vi "Prod_Screen.vi"(1 "gain_in":dbl format="%#_13g", 2 "nf_in":dbl format="%#_13g", 3 "pow_in":dbl format="%#_13g", 5 "error in (no error)":errorcluster, 7 "s11_in":dbl format="%#_13g", 9 "txflat_in":dbl format="%#_13g", 11 "pout_in":dbl format="%#_13g") -> (6 "rx_p-f":string, 8 "tx_p-f":string, 10 "RX-PASS?(T)":bool, 12 "TX-PASS?(T)":bool, 15 "prod_lim_p-f":string, 19 "error out":errorcluster)   [LabVIEW 2018]
uses:
  Tetra_Globals.vi
panel:
  out "gain_lsl":dbl
  out "names 10":string
  out "end":bool
  out "pout_pass?(t)":bool
  out "tx-flat_pass?(t)":bool
  out "s11_pass?(t)":bool
  out "pow_pass?(t)":bool
  out "nf_pass?(t)":bool
  out "gain_pass?(t)":bool
  out "names 9":string
  out "limits 9":dbl
  out "names 8":string
  out "limits 8":dbl
  out "names 7":string
  out "pout_hsl":dbl
  out "names 6":string
  out "pout_lsl":dbl
  out "names 5":string
  out "txflat":dbl
  out "names 4":string
  out "s11_hsl":dbl
  out "names 3":string
  out "pow_hsl":dbl
  out "names 2":string
  out "nf_hsl":dbl
  out "gain_hsl":dbl
  out "names":string
  # "pdc|g|nf"
  # "pdc|s11|txf|txp"
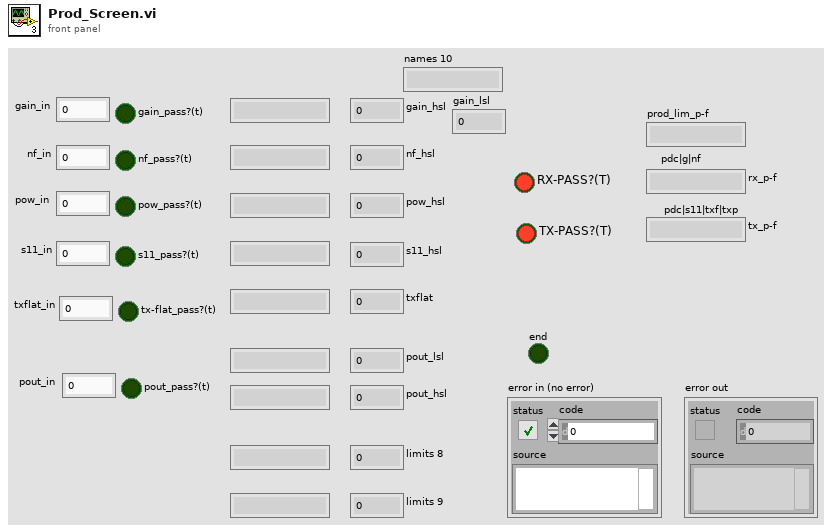
[diagram p1: front panel]
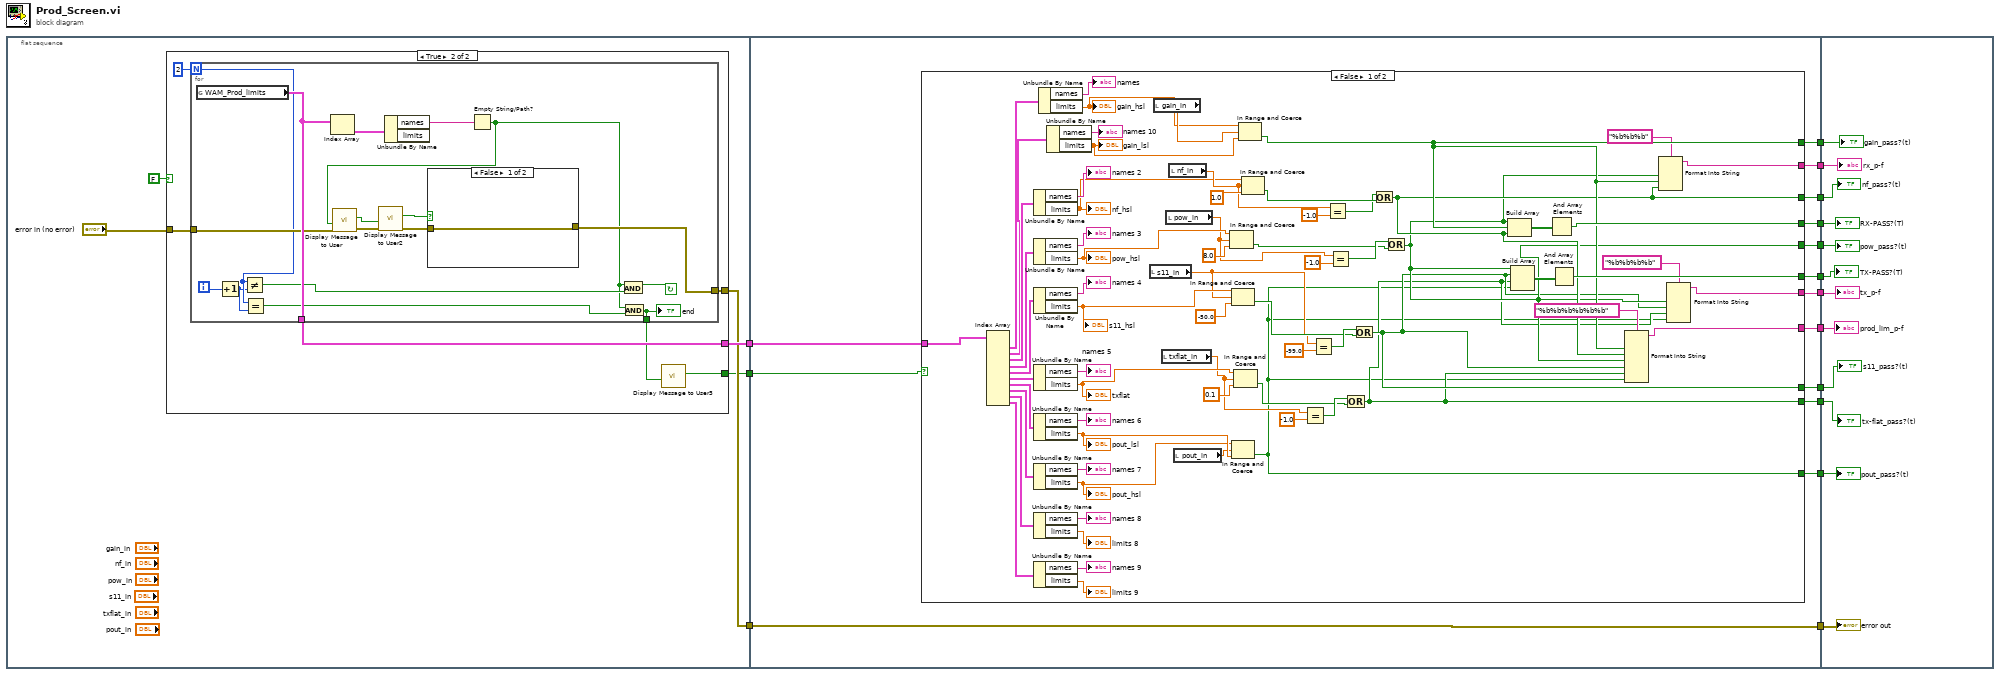
[diagram p0: block diagram]
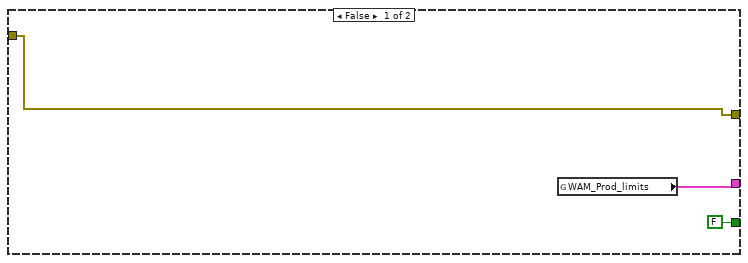
[diagram p2: hidden frame]
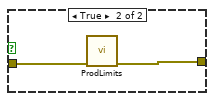
[diagram p3: hidden frame]
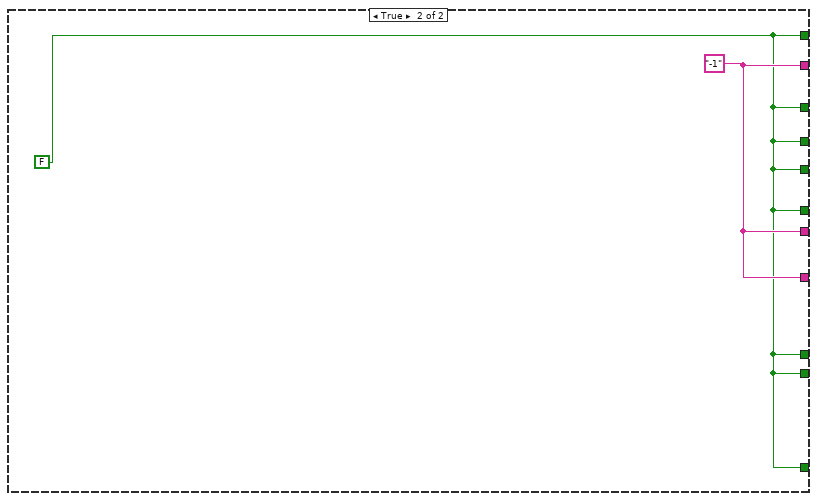
[diagram p4: hidden frame]
diagram:
  n1 = flat-sequence {
    tunnel: [w20] -> w15
    tunnel: [w18] -> w13
    tunnel: [w17] -> w12
    tunnel: w15 -> [w63]
    tunnel: [w62] -> w14
    tunnel: w13 -> [w62]
    tunnel: w12 -> [w61]
    tunnel: [w60] -> w11
    tunnel: [w59] -> w10
    tunnel: [w58] -> w9
    tunnel: [w57] -> w8
    tunnel: [w56] -> w7
    tunnel: [w55] -> w6
    tunnel: [w54] -> w5
    tunnel: [w53] -> w4
    tunnel: [w52] -> w3
    tunnel: [w51] -> w2
    tunnel: [w50] -> w1
    tunnel: w14 -> [w146]
    tunnel: w11 -> [w145]
    tunnel: w10 -> [w144]
    tunnel: w9 -> [w143]
    tunnel: w8 -> [w142]
    tunnel: w7 -> [w141]
    tunnel: w6 -> [w140]
    tunnel: w5 -> [w139]
    tunnel: w4 -> [w138]
    tunnel: w3 -> [w137]
    tunnel: w2 -> [w136]
    tunnel: w1 -> [w135]
    frame #0 {
      n2 = case shown="True" FALSE {
        tunnel: [w23 w29] -> w20
        tunnel: "error in (no error)" -> [w21 w27]
        tunnel: [w21 w26] -> w18
        tunnel: [FALSE ("OK") w24] -> w17
        frame False {
          n3 = global read "Tetra_Globals.vi" "WAM_Prod_limits"() -> (w23:cluster{"names":string, "limits":dbl}[])
        }
        frame True {
          n4 = for {
            N: 2 -> [w33]
            tunnel: [w46] -> w29
            tunnel: w27 -> [w38]
            tunnel: [w37] -> w26
            tunnel: [w30] -> w25
            i -> [w39]
            stop <- w36 continue-if-true
            n5 = global read "Tetra_Globals.vi" "WAM_Prod_limits"() -> (w46:cluster{"names":string, "limits":dbl}[])
            n6 = Increment(x=w39) -> (x+1=w32:i32)
            n7 = Not Equal?(x=w33, y=w32) -> (x != y?=w35:bool)
            n8 = Equal?(x=w33, y=w32) -> (x = y?=w31:bool)
            n9 = Index Array(array=w46) -> (element=w45:cluster{"names":string, "limits":dbl})  [unwired: 1 in]
            n10 = Unbundle By Name(w45) -> ("names"=w44:string)  [unwired: 1 out]
            n11 = Empty String/Path?(string/path=w44) -> (empty?=w34:bool)
            n12 = call "Display Message to User"("error in (no error)"=w38, "Enable"=w34) -> ("error out"=w41:errorcluster, "OK"=w42:bool)  [unwired: 8 in]
            n13 = call "Display Message to User2"("error in (no error)"=w41, "Enable"=w42) -> ("error out"=w40:errorcluster, "OK"=w43:bool)  [unwired: 8 in]
            n14 = case shown="False" w43 {
              tunnel: w40 -> [w47 w49]
              tunnel: [w47 w48] -> w37
              frame False {
              }
              frame True {
                n15 = call "ProdLimits.vi"("error in (no error)"=w49) -> ("error out"=w48:errorcluster)  [unwired: 9 in, 1 out]
              }
            }
            n16 = And(x=w34, y=w35) -> (x .and. y?=w36:bool)
            n17 = And(x=w34, y=w31) -> (x .and. y?=w30:bool)
            "end" <- w30
          }
          n18 = call "Display Message to User3"("Enable"=w25) -> ("OK"=w24:bool)  [unwired: 9 in, 1 out]
        }
      }
    }
    frame #1 {
      n19 = case shown="False" w61 {
        tunnel: w63 -> [w132 _]
        tunnel: [w80 w133] -> w60
        tunnel: [w79 w133] -> w59
        tunnel: [w83 w133] -> w58
        tunnel: [w74 w133] -> w57
        tunnel: [w82 w133] -> w56
        tunnel: [w81 w134] -> w55
        tunnel: [w73 w133] -> w54
        tunnel: [w72 w133] -> w53
        tunnel: [w71 w133] -> w52
        tunnel: [w78 w134] -> w51
        tunnel: [w75 w134] -> w50
        frame False {
          n20 = Index Array(array=w132) -> (element #1=w69:cluster{"names":string, "limits":dbl}, element #2=w66:cluster{"names":string, "limits":dbl}, element #3=w67:cluster{"names":string, "limits":dbl}, element #4=w129:cluster{"names":string, "limits":dbl}, element #5=w120:cluster{"names":string, "limits":dbl}, element #6=w119:cluster{"names":string, "limits":dbl}, element #7=w118:cluster{"names":string, "limits":dbl}, element #8=w117:cluster{"names":string, "limits":dbl}, element #9=w116:cluster{"names":string, "limits":dbl}, element #10=w115:cluster{"names":string, "limits":dbl})  [unwired: 10 in]
          n21 = Unbundle By Name(w67) -> ("names"=→"names 2":string, "limits"=w68:dbl)
          "nf_hsl" <- w68
          n22 = Unbundle By Name(w129) -> ("names"=→"names 3":string, "limits"=w112:dbl)
          "pow_hsl" <- w112
          n23 = Unbundle By Name(w120) -> ("names"=→"names 4":string, "limits"=w110:dbl)
          "s11_hsl" <- w110
          n24 = Unbundle By Name(w119) -> ("names"=→"names 5":string, "limits"=w109:dbl)
          "txflat" <- w109
          n25 = Unbundle By Name(w118) -> ("names"=→"names 6":string, "limits"=w107:dbl)
          "pout_lsl" <- w107
          n26 = Unbundle By Name(w117) -> ("names"=→"names 7":string, "limits"=w106:dbl)
          "pout_hsl" <- w106
          n27 = Unbundle By Name(w116) -> ("names"=→"names 8":string, "limits"=→"limits 8":dbl)
          n28 = Unbundle By Name(w115) -> ("names"=→"names 9":string, "limits"=→"limits 9":dbl)
          n29 = Unbundle By Name(w69) -> ("names"=→"names":string, "limits"=w70:dbl)
          "gain_hsl" <- w70
          n30 = Unbundle By Name(w66) -> ("names"=→"names 10":string, "limits"=w64:dbl)
          "gain_lsl" <- w64
          n31 = local read "s11_in"() -> (w87:dbl)
          n32 = local read "gain_in"() -> (w90:dbl)
          n33 = local read "txflat_in"() -> (w86:dbl)
          n34 = local read "pow_in"() -> (w88:dbl)
          n35 = local read "nf_in"() -> (w89:dbl)
          n36 = local read "pout_in"() -> (w85:dbl)
          n37 = In Range and Coerce(upper limit=w112, x=w88, lower limit=8.0) -> (In Range?=w98:bool)  [unwired: 1 out]
          n38 = In Range and Coerce(upper limit=w110, x=w87, lower limit=-50.0) -> (In Range?=w95:bool)  [unwired: 1 out]
          n39 = In Range and Coerce(upper limit=w106, x=w85, lower limit=w107) -> (In Range?=w71:bool)  [unwired: 1 out]
          n40 = In Range and Coerce(upper limit=w109, x=w86, lower limit=0.1) -> (In Range?=w92:bool)  [unwired: 1 out]
          n41 = In Range and Coerce(upper limit=w70, x=w90, lower limit=w64) -> (In Range?=w80:bool)  [unwired: 1 out]
          n42 = In Range and Coerce(upper limit=w68, x=w89, lower limit=1.0 ("upper limit")) -> (In Range?=w103:bool)  [unwired: 1 out]
          n43 = Equal?(x=w86, y=-1.0) -> (x = y?=w93:bool)
          n44 = Equal?(x=w87, y=-99.0) -> (x = y?=w97:bool)
          n45 = Equal?(x=w89, y=-1.0) -> (x = y?=w102:bool)
          n46 = Equal?(x=w88, y=-1.0) -> (x = y?=w99:bool)
          n47 = Or(x=w93, y=w92) -> (x .or. y?=w72:bool)
          n48 = Or(x=w97, y=w95) -> (x .or. y?=w73:bool)
          n49 = Or(x=w102, y=w103) -> (x .or. y?=w79:bool)
          n50 = Or(x=w99, y=w98) -> (x .or. y?=w74:bool)
          n51 = Build Array(w74, w80, w79) -> (w104:bool[])
          n52 = Build Array(w74, w73, w72, w71) -> (w105:bool[])
          n53 = And Array Elements(Boolean array=w104) -> (logical AND=w83:bool)
          n54 = And Array Elements(Boolean array=w105) -> (logical AND=w82:bool)
          n55 = Format Into String(format string="%b%b%b%b%b%b", w80, w79, w74, w73, w72, w71) -> (resulting string=w81:string)  [unwired: 2 in, 1 out]
          n56 = Format Into String(format string="%b%b%b", w74, w80, w79) -> (resulting string=w78:string)  [unwired: 2 in, 1 out]
          n57 = Format Into String(format string="%b%b%b%b", w74, w73, w72, w71) -> (resulting string=w75:string)  [unwired: 2 in, 1 out]
        }
        frame True {
          w134 = "-1"
          w133 = FALSE ("nf_pass?(t)")
        }
      }
    }
    frame #2 {
      "error out" <- w146
      "gain_pass?(t)" <- w145
      "nf_pass?(t)" <- w144
      "RX-PASS?(T)" <- w143
      "pow_pass?(t)" <- w142
      "TX-PASS?(T)" <- w141
      "prod_lim_p-f" <- w140
      "s11_pass?(t)" <- w139
      "tx-flat_pass?(t)" <- w138
      "pout_pass?(t)" <- w137
      "rx_p-f" <- w136
      "tx_p-f" <- w135
    }
  }
